vi "Main VI.vi"() -> ()   [LabVIEW 2016]
doc: "Tile child windows in MDI panel"
uses:
  source code/MDI Library/TypeDefs/Set Position.ctl
  Typedef/Queue Operation.ctl
  Typedef/Main VI Data Cluster.ctl
  source code/MDI Library/LV MDI.lvclass
  source code/Document/Document.lvclass
  <vilib>/Utility/error.llb/DialogType.ctl
  source code/MDI Library/Public/Create.vi
  source code/MDI Library/Public/Add.vi
  source code/MDI Library/Public/Remove.vi
  source code/MDI Library/Public/Set Position.vi
  source code/MDI Library/Public/Show.vi
  source code/MDI Library/Public/Hide.vi
  source code/MDI Library/Public/Save.vi
  source code/MDI Library/Public/Recall.vi
  source code/MDI Library/Public/Dock.vi
  source code/MDI Library/Public/Tile.vi
  source code/MDI Library/Public/Cascade.vi
  source code/MDI Library/Public/Destroy.vi
  user32.dll
  System.Windows.Forms
  source code/Document/Child Classes/Py Doc/Py Doc.lvclass
  source code/Document/Child Classes/LV Doc/Child Classes/LV DEV/LV DEV.lvclass
panel:
  in  "Py File Path":path
  in  "XML File Path":path
  in  "Recall":bool
  in  "Save":bool
  in  "Position[]":T1[](array[typedef]) caption="Set Position for selected Documents"
  in  "Remove":bool
  in  "Cascade & Order":cluster{"Order":u16, "Cascade":bool}={"Order"=2, "Cascade"=FALSE} {"Order" items=["List order"=2, "Z order"=4]}
  in  "Tile & Direction":cluster{"Direction":u16, "Tile":bool} {"Direction" items=["Vertical", "Horizontal"]}
  in  "Listbox":i32[](listbox)
  in  "Undock":bool
  in  "Add":bool
  in  "Hide":bool
  in  "Show":bool
  in  "Stop":bool
  in  "LV Dev Path":path
  in  "Container":refnum<k24>(container)
  out "Error Out":errorcluster
  in  "Error In":errorcluster
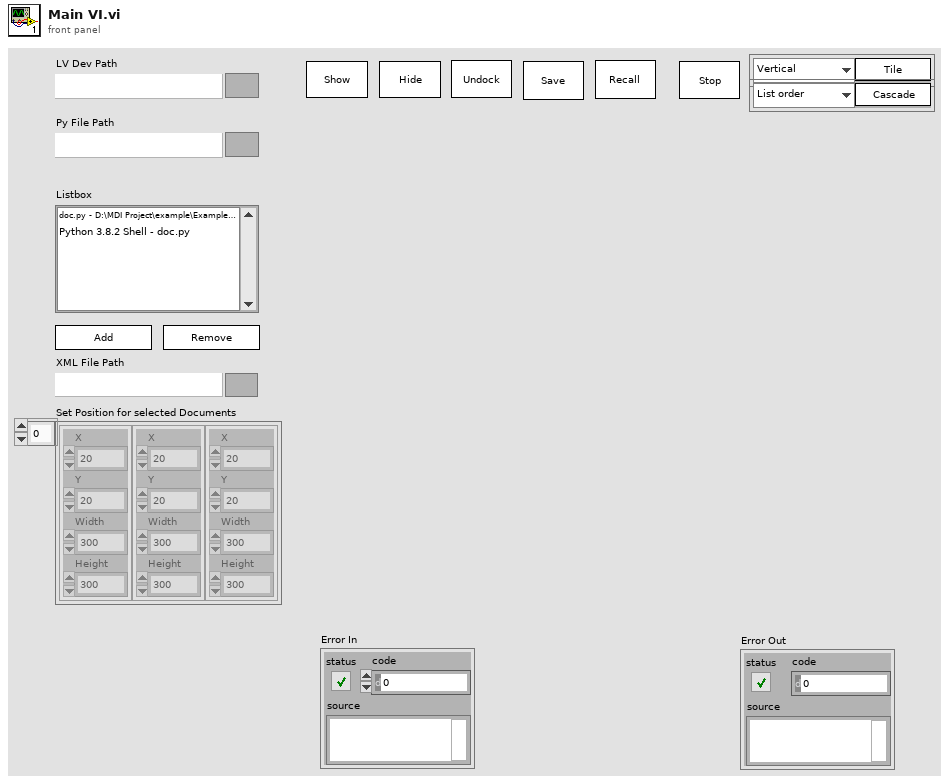
[diagram p1: front panel]
types:
  T1 = typedef "LV MDI.lvclass/Set Position.ctl" = cluster{"X":i32, "Y":i32, "Width":i32, "Height":i32}
  T2 = typedef "Queue Operation.ctl" = enum16{"Create Queue", "Enqueue N Element", "Enstack N Element", "Dequeue 1 Element", "Flush Queue", "Close Queue"}
  T3 = typedef "Main VI Data Cluster.ctl" = cluster{"MDI Object":refnum<class "LV MDI.lvclass">, "Container Refnum":refnum<k24>, "LV Dev  Path":path, "Document Name[]":string[], "LV hwnd":u32, "Dock?":bool, "Position[] ":T1[], "XML File Path ":path, "Document Class":refnum<class "Document.lvclass">, "Py file Path":path, "Document Class[]":refnum<class "Document.lvclass">[]}
  T4 = typedef "DialogType.ctl" = u16
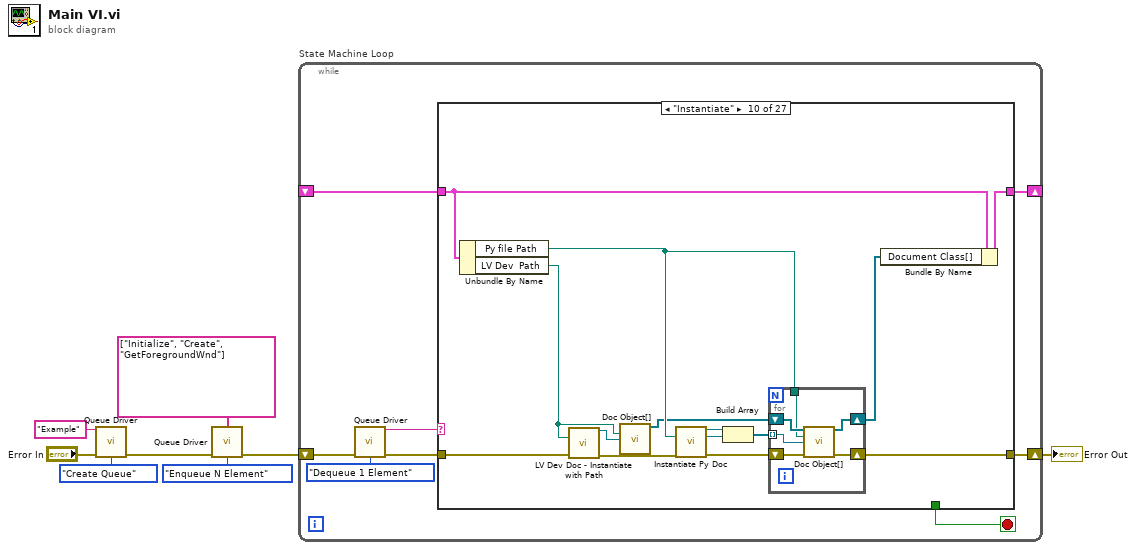
[diagram p0: block diagram]
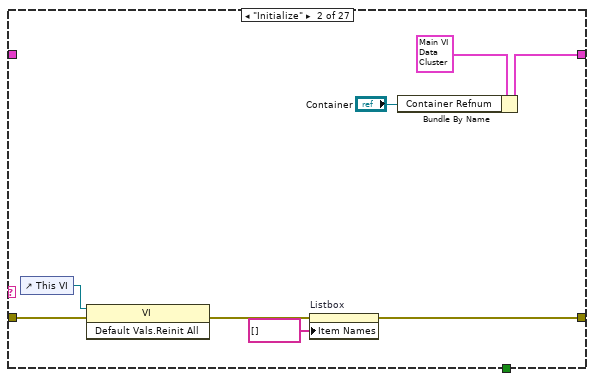
[diagram p3: hidden frame]
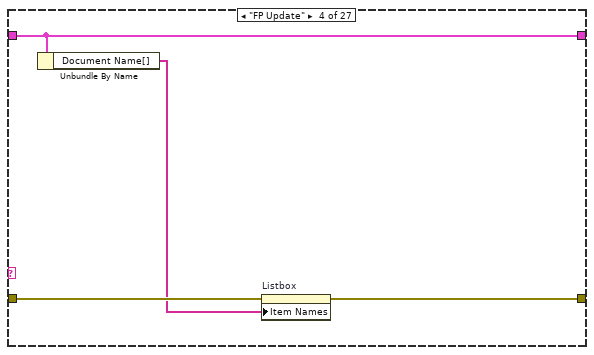
[diagram p5: hidden frame]
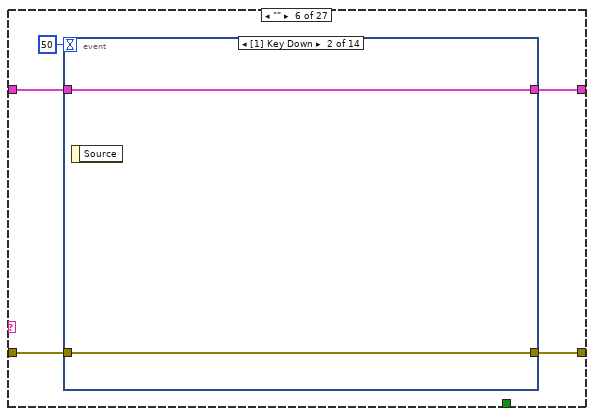
[diagram p7: hidden frame]
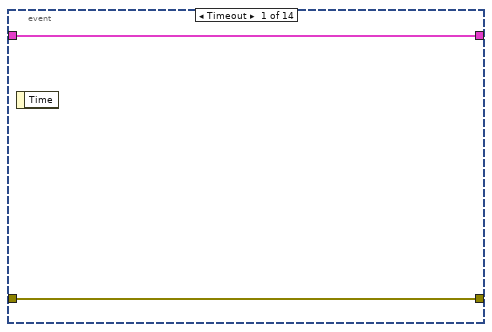
[diagram p8: hidden frame]
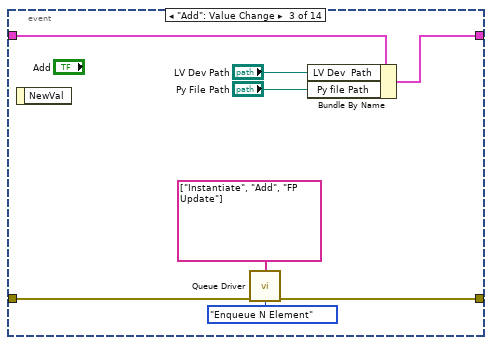
[diagram p9: hidden frame]
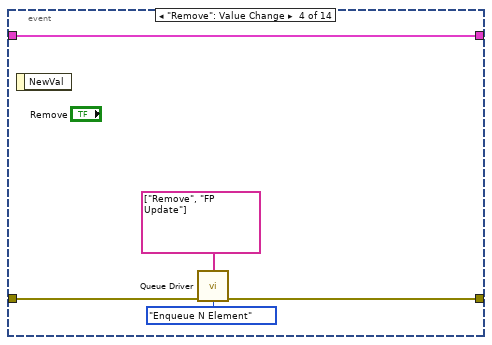
[diagram p10: hidden frame]
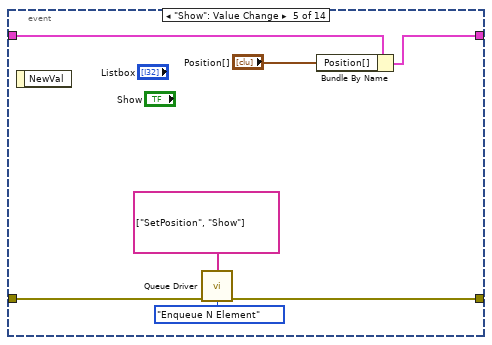
[diagram p11: hidden frame]
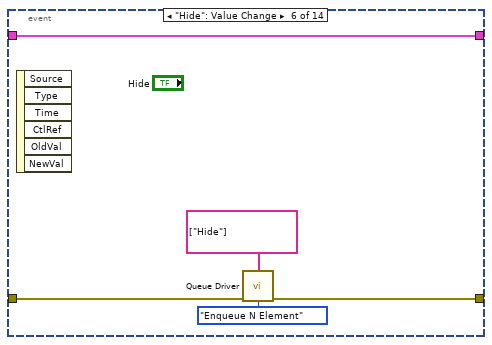
[diagram p12: hidden frame]
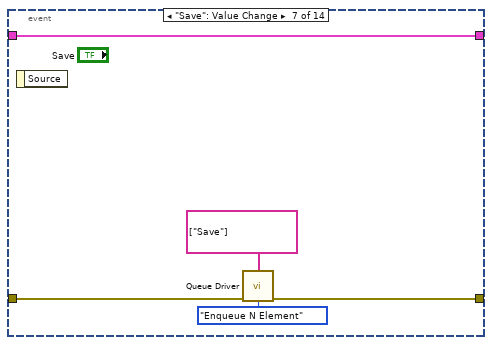
[diagram p13: hidden frame]
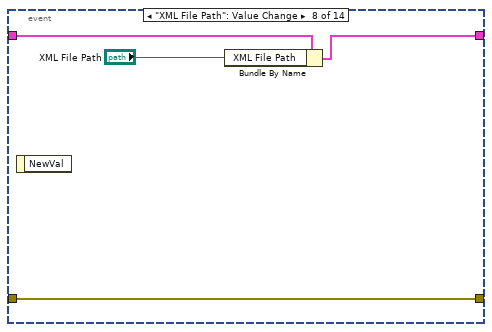
[diagram p14: hidden frame]
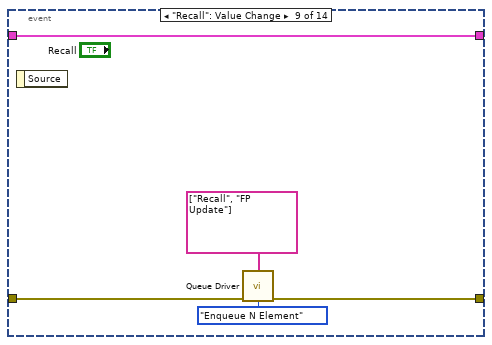
[diagram p15: hidden frame]
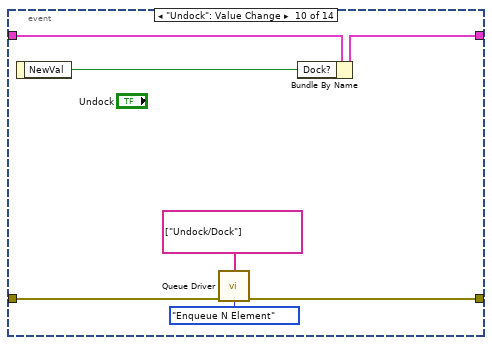
[diagram p16: hidden frame]
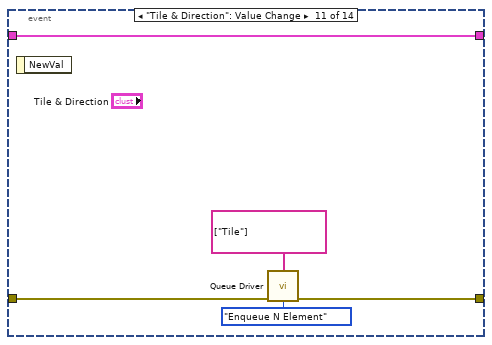
[diagram p17: hidden frame]
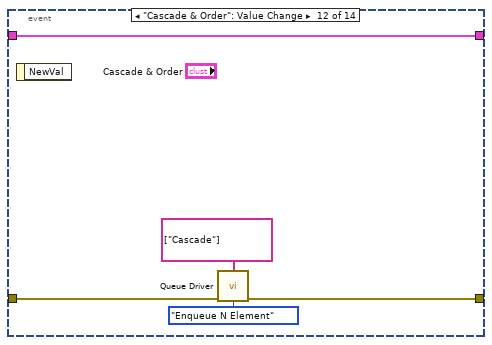
[diagram p18: hidden frame]
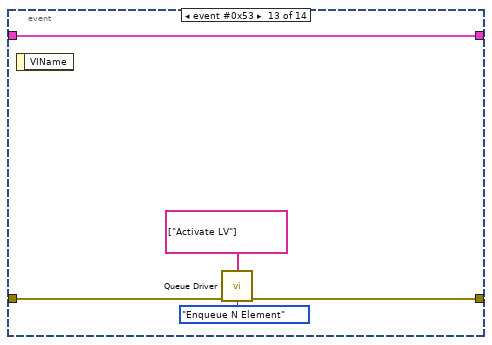
[diagram p19: hidden frame]
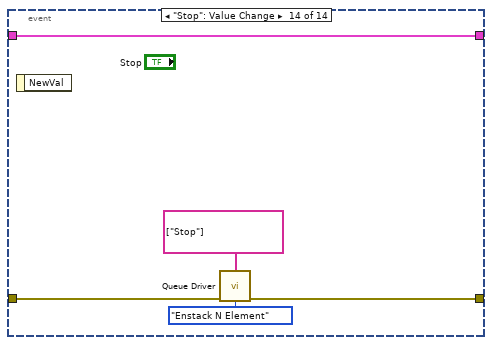
[diagram p20: hidden frame]
diagram:
  n1 = call "Queue Driver.vi"("Queue Name"="Example", "error In"="Error In", "Queue Operation"=Queue_Operation."Create Queue") -> ("error out"=w6:errorcluster)  [unwired: 11 in, 1 out]
  n2 = call "Queue Driver.vi"("States[]"=string[] ["Initialize", "Create", "GetForegroundWnd"], "error In"=w6, "Queue Operation"=Queue_Operation."Enqueue N Element") -> ("error out"=w3:errorcluster)  [unwired: 11 in, 1 out]
  n3 = while "State Machine Loop" {
    shift-right: [w15] -> w7
    shift-left: w3 -> [w16]
    shift-right: [w10] -> _
    shift-left: _ -> [w9]
    stop <- w11 stop-if-true
    n4 = call "Queue Driver.vi"("error In"=w16, "Queue Operation"=Queue_Operation."Dequeue 1 Element") -> ("Dequeued State"=w12:string, "error out"=w14:errorcluster)  [unwired: 12 in]
    n5 = case shown="\"Instantiate\"" w12 {
      selector: w12 -> [_ _ _ _ _ _ _ _ _ _ _ _ _ _ _ _ _ _ _ _ _ _ _ _ w258 _ _]
      tunnel: w14 -> [w18 w26 w28 w32 w34 w39 w111 w118 w123 w128 w149 w167 w172 w186 w190 w202 w209 w221 w223 w231 w239 w241 w245 w251 w259 w272 w284]
      tunnel: [w18 w20 w28 w31 w34 w38 w111 w117 w122 w134 w148 w161 w177 w185 w195 w201 w208 w220 w223 w230 w238 w241 w244 w251 w255 w262 w290] -> w15
      tunnel: [_ _ _ _ _ _ _ _ _ _ _ _ _ _ _ _ _ _ _ _ _ _ _ _ _ _ TRUE] -> w11
      tunnel: [w17 w24 w27 w30 w33 w35 w110 w114 w120 w136 w150 w164 w174 w181 w192 w198 w210 w217 w222 w226 w234 w240 w243 w250 w252 w260 w287] -> w10
      tunnel: w9 -> [w17 _ w27 w30 w33 w36 w110 w115 w121 w137 w151 w165 w175 w182 w193 w199 w211 w218 w222 w227 w235 w240 w243 w250 w252 w260 w288]
      frame "----------------------Initialization---------------------" {
      }
      frame "Initialize" {
        n6 = control-ref of="This VI"() -> (w21:refnum<vi>)
        n7 = invoke class="VI" method="Default Vals.Reinit All"(reference=w21, error in=w26) -> (error out=w22:errorcluster)  [unwired: 1 in, 2 out]
        n8 = property on="Listbox" class="LstBox (strict)"(error in=w22, "Item Names"=string[] []) -> (error out=w20:errorcluster)  [unwired: 1 in, 1 out]
        n9 = Bundle By Name(cluster=T3 {"MDI Object"=refnum, "Container Refnum"=refnum, "LV Dev  Path"=path "", "Document Name[]"=[], "LV hwnd"=0, "Dock?"=FALSE, "Position[] "=[], "XML File Path "=path "", "Document Class"=refnum, "Py file Path"=path "", "Document Class[]"=[]}, "Container Refnum"="Container") -> (w24:T3)
      }
      frame "----------------------Front Panel Update-------------" {
      }
      frame "FP Update" {
        n10 = Unbundle By Name(w30) -> ("Document Name[]"=w29:string[])
        n11 = property on="Listbox" class="LstBox (strict)"(error in=w32, "Item Names"=w29) -> (error out=w31:errorcluster)  [unwired: 1 in, 1 out]
      }
      frame "----------------------Poll-------------------------------" {
      }
      frame "" {
        n12 = event shown="[1] Key Down" {
          selector: _ -> [_ _ _ _ _ _ _ _ _ _ _ _ _ _]
          dyn-events: _ -> [_ _ _ _ _ _ _ _ _ _ _ _ _ _]
          timeout: 50 -> [_ _ _ _ _ _ _ _ _ _ _ _ _ _]
          tunnel: [w41 w43 w47 w54 w62 w66 w72 w77 w80 w88 w92 w97 w102 w107] -> w38
          tunnel: w39 -> [w41 w43 w51 w56 w63 w68 w73 w77 w82 w89 w94 w99 w104 w109]
          tunnel: [w40 w42 w48 w55 w58 w67 w69 w75 w81 w84 w93 w98 w103 w108] -> w35
          tunnel: w36 -> [w40 w42 w49 w55 w59 w67 w69 w76 w81 w85 w93 w98 w103 w108]
          event Timeout {
            n13 = event-data() -> ()  [unwired: 1 in, 1 out]
          }
          event Key Down {
            n14 = event-data() -> ()  [unwired: 1 in, 1 out]
          }
          event "Add": Value Change {
            n15 = event-data() -> ()  [unwired: 1 in, 1 out]
            n16 = call "Queue Driver.vi"("States[]"=string[] ["Instantiate", "Add", "FP Update"], "error In"=w51, "Queue Operation"=Queue_Operation."Enqueue N Element") -> ("error out"=w47:errorcluster)  [unwired: 11 in, 1 out]
            n17 = Bundle By Name(cluster=w49, "LV Dev  Path"="LV Dev Path", "Py file Path"="Py File Path") -> (w48:T3)
          }
          event "Remove": Value Change {
            n18 = event-data() -> ()  [unwired: 1 in, 1 out]
            n19 = call "Queue Driver.vi"("States[]"=string[] ["Remove", "FP Update"], "error In"=w56, "Queue Operation"=Queue_Operation."Enqueue N Element") -> ("error out"=w54:errorcluster)  [unwired: 11 in, 1 out]
          }
          event "Show": Value Change {
            n20 = event-data() -> ()  [unwired: 1 in, 1 out]
            n21 = call "Queue Driver.vi"("States[]"=string[] ["SetPosition", "Show"], "error In"=w63, "Queue Operation"=Queue_Operation."Enqueue N Element") -> ("error out"=w62:errorcluster)  [unwired: 11 in, 1 out]
            n22 = Bundle By Name(cluster=w59, "Position[]"="Position[]") -> (w58:T3)
          }
          event "Hide": Value Change {
            n23 = event-data() -> ()  [unwired: 1 in, 6 out]
            n24 = call "Queue Driver.vi"("States[]"=string[] ["Hide"], "error In"=w68, "Queue Operation"=Queue_Operation."Enqueue N Element") -> ("error out"=w66:errorcluster)  [unwired: 11 in, 1 out]
          }
          event "Save": Value Change {
            n25 = event-data() -> ()  [unwired: 1 in, 1 out]
            n26 = call "Queue Driver.vi"("States[]"=string[] ["Save"], "error In"=w73, "Queue Operation"=Queue_Operation."Enqueue N Element") -> ("error out"=w72:errorcluster)  [unwired: 11 in, 1 out]
          }
          event "XML File Path": Value Change {
            n27 = event-data() -> ()  [unwired: 1 in, 1 out]
            n28 = Bundle By Name(cluster=w76, "XML File Path"="XML File Path") -> (w75:T3)
          }
          event "Recall": Value Change {
            n29 = event-data() -> ()  [unwired: 1 in, 1 out]
            n30 = call "Queue Driver.vi"("States[]"=string[] ["Recall", "FP Update"], "error In"=w82, "Queue Operation"=Queue_Operation."Enqueue N Element") -> ("error out"=w80:errorcluster)  [unwired: 11 in, 1 out]
          }
          event "Undock": Value Change {
            n31 = event-data() -> ("NewVal"=w83:bool)  [unwired: 1 in]
            n32 = call "Queue Driver.vi"("States[]"=string[] ["Undock/Dock"], "error In"=w89, "Queue Operation"=Queue_Operation."Enqueue N Element") -> ("error out"=w88:errorcluster)  [unwired: 11 in, 1 out]
            n33 = Bundle By Name(cluster=w85, "Dock?"=w83) -> (w84:T3)
          }
          event "Tile & Direction": Value Change {
            n34 = event-data() -> ()  [unwired: 1 in, 1 out]
            n35 = call "Queue Driver.vi"("States[]"=string[] ["Tile"], "error In"=w94, "Queue Operation"=Queue_Operation."Enqueue N Element") -> ("error out"=w92:errorcluster)  [unwired: 11 in, 1 out]
          }
          event "Cascade & Order": Value Change {
            n36 = event-data() -> ()  [unwired: 1 in, 1 out]
            n37 = call "Queue Driver.vi"("States[]"=string[] ["Cascade"], "error In"=w99, "Queue Operation"=Queue_Operation."Enqueue N Element") -> ("error out"=w97:errorcluster)  [unwired: 11 in, 1 out]
          }
          event event #0x53 {
            n38 = event-data() -> ()  [unwired: 1 in, 1 out]
            n39 = call "Queue Driver.vi"("States[]"=string[] ["Activate LV"], "error In"=w104, "Queue Operation"=Queue_Operation."Enqueue N Element") -> ("error out"=w102:errorcluster)  [unwired: 11 in, 1 out]
          }
          event "Stop": Value Change {
            n40 = event-data() -> ()  [unwired: 1 in, 1 out]
            n41 = call "Queue Driver.vi"("States[]"=string[] ["Stop"], "error In"=w109, "Queue Operation"=Queue_Operation."Enstack N Element") -> ("error out"=w107:errorcluster)  [unwired: 11 in, 1 out]
          }
        }
      }
      frame "----------------------MDI API-------------------------" {
      }
      frame "Create" {
        n42 = Unbundle By Name(w115) -> ("MDI Object"=w116:refnum<class "LV MDI.lvclass">, "Container Refnum"=w112:refnum<k24>)
        n43 = call-poly "MDI.vi"("LV MDI in"=w116, "Panel Reference"=w112, "error in (no error)"=w118) -> ("LV MDI out"=w113:refnum<class "LV MDI.lvclass">, "error out"=w117:errorcluster)  [unwired: 11 in]
        n44 = Bundle By Name(cluster=w115, "MDI Object"=w113) -> (w114:T3)
      }
      frame "GetForegroundWnd" {
        n45 = dll-call lib="user32.dll" fn="GetForegroundWindow"(error in=w123) -> (error out=w122:errorcluster, "hwnd"=w119:u32)  [unwired: 2 in, 1 out]
        n46 = Bundle By Name(cluster=w121, "LV hwnd"=w119) -> (w120:T3)
      }
      frame "Instantiate" {
        n47 = Unbundle By Name(w137) -> ("Py file Path"=w132:path, "LV Dev  Path"=w124:path)
        n48 = call "LV Dev Doc - Instantiate with Path.vi"("LV Doc Path"=w124, "error in (no error)"=w128) -> ("Document out"=w125:refnum<class "Document.lvclass">, "error out"=w127:errorcluster)  [unwired: 12 in]
        n49 = call "Doc Object[].vi"("Path"=w124, "Document Class"=w125) -> ("Document Class[]"=w126:refnum<class "Document.lvclass">[])  [unwired: 12 in, 1 out]
        n50 = call "Instantiate Py Doc.vi"("Py File Path"=w132, "error in (no error)"=w127) -> ("Editor Document"=w131:refnum<class "Document.lvclass">, "Shell Document"=w130:refnum<class "Document.lvclass">, "error out"=w133:errorcluster)  [unwired: 11 in]
        n51 = Build Array(w131, w130) -> (w129:refnum<class "Document.lvclass">[])
        n52 = for {
          tunnel: w132 -> [w139]
          shift-right: [w143] -> w135
          shift-left: w126 -> [w142]
          shift-right: [w141] -> w134
          shift-left: w133 -> [w140]
          tunnel: w129 -> [w138] mode=indexing
          n53 = call "Doc Object[].vi"("Document Class[]"=w142, "Path"=w139, "Document Class"=w138, "error in (no error)"=w140) -> ("Document Class[]"=w143:refnum<class "Document.lvclass">[], "error out"=w141:errorcluster)  [unwired: 10 in]
        }
        n54 = Bundle By Name(cluster=w137, "Document Class[]"=w135) -> (w136:T3)
      }
      frame "Add" {
        n55 = Unbundle By Name(w151) -> ("MDI Object"=w147:refnum<class "LV MDI.lvclass">, "Document Class[]"=w144:refnum<class "Document.lvclass">[])
        n56 = for {
          tunnel: [w153] -> w145
          shift-right: [w156] -> w148
          shift-left: w149 -> [w157]
          shift-right: [w154] -> w146
          shift-left: w147 -> [w155]
          tunnel: w144 -> [w152] mode=indexing
          n57 = call-poly "MDI.vi"("LV MDI.lvclass"=w155, "Document class"=w152, "error in (no error)"=w157) -> ("LV MDI.lvclass"=w154:refnum<class "LV MDI.lvclass">, "Name[]"=w153:string[], "error out"=w156:errorcluster)  [unwired: 10 in]
        }
        n58 = Bundle By Name(cluster=w151, "MDI Object"=w146, "Document Name[]"=w145) -> (w150:T3)
      }
      frame "Remove" {
        n59 = Unbundle By Name(w165) -> ("MDI Object"=w166:refnum<class "LV MDI.lvclass">)
        n60 = control-ref of="Listbox"() -> (w159:refnum<vi>)
        n61 = call "Selected Doc Name[].vi"("error in (no error)"=w167, "ListBox in"=w159) -> ("error out"=w162:errorcluster, "Array"=w160:string[])  [unwired: 8 in]
        n62 = call-poly "MDI.vi"("LV MDI in"=w166, "Doc Name[]"=w160, "error in (no error)"=w162) -> ("LV MDI out"=w163:refnum<class "LV MDI.lvclass">, "Doc Name out[]"=w158:string[], "error out"=w161:errorcluster)  [unwired: 10 in]
        n63 = Bundle By Name(cluster=w165, "MDI Object"=w163, "Document Name[]"=w158) -> (w164:T3)
      }
      frame "SetPosition" {
        n64 = control-ref of="Listbox"() -> (w169:refnum<vi>)
        n65 = Unbundle By Name(w175) -> ("MDI Object"=w176:refnum<class "LV MDI.lvclass">, "Position[]"=w168:T1[])
        n66 = call "Selected Doc Name[].vi"("error in (no error)"=w172, "ListBox in"=w169) -> ("error out"=w171:errorcluster, "Array"=w170:string[])  [unwired: 8 in]
        n67 = call-poly "MDI.vi"("LV MDI.lvclass"=w176, "Position[]"=w168, "Doc Name[]"=w170, "error in (no error)"=w171) -> ("LV MDI.lvclass"=w173:refnum<class "LV MDI.lvclass">, "error out"=w177:errorcluster)  [unwired: 10 in]
        n68 = Bundle By Name(cluster=w175, "MDI Object"=w173) -> (w174:T3)
      }
      frame "Show" {
        n69 = control-ref of="Listbox"() -> (w178:refnum<vi>)
        n70 = Unbundle By Name(w182) -> ("MDI Object"=w184:refnum<class "LV MDI.lvclass">)
        n71 = call "Selected Doc Name[].vi"("error in (no error)"=w186, "ListBox in"=w178) -> ("error out"=w180:errorcluster, "Array"=w179:string[])  [unwired: 8 in]
        n72 = call-poly "MDI.vi"("LV MDI in"=w184, "Doc Name[]"=w179, "error in (no error)"=w180) -> ("LV MDI out"=w183:refnum<class "LV MDI.lvclass">, "error out"=w185:errorcluster)  [unwired: 11 in]
        n73 = Bundle By Name(cluster=w182, "MDI Object"=w183) -> (w181:T3)
      }
      frame "Hide" {
        n74 = control-ref of="Listbox"() -> (w187:refnum<vi>)
        n75 = Unbundle By Name(w193) -> ("MDI Object"=w194:refnum<class "LV MDI.lvclass">)
        n76 = call "Selected Doc Name[].vi"("error in (no error)"=w190, "ListBox in"=w187) -> ("error out"=w189:errorcluster, "Array"=w188:string[])  [unwired: 8 in]
        n77 = call-poly "MDI.vi"("LV MDI in"=w194, "Doc Name[]"=w188, "error in (no error)"=w189) -> ("LV MDI out"=w191:refnum<class "LV MDI.lvclass">, "error out"=w195:errorcluster)  [unwired: 11 in]
        n78 = Bundle By Name(cluster=w193, "MDI Object"=w191) -> (w192:T3)
      }
      frame "Save" {
        n79 = Unbundle By Name(w199) -> ("MDI Object"=w200:refnum<class "LV MDI.lvclass">, "XML File Path"=w196:path)
        n80 = call-poly "MDI.vi"("LV MDI in"=w200, "XML File Path"=w196, "error in (no error)"=w202) -> ("LV MDI out"=w197:refnum<class "LV MDI.lvclass">, "error out"=w201:errorcluster)  [unwired: 11 in]
        n81 = Bundle By Name(cluster=w199, "MDI Object"=w197) -> (w198:T3)
      }
      frame "Recall" {
        n82 = Unbundle By Name(w211) -> ("MDI Object"=w206:refnum<class "LV MDI.lvclass">, "XML File Path"=w205:path, "Container Refnum"=w204:refnum<k24>)
        n83 = call-poly "MDI.vi"("LV MDI in"=w206, "XML File Path"=w205, "Container Refnum"=w204, "error in (no error)"=w209) -> ("LV MDI out"=w207:refnum<class "LV MDI.lvclass">, "Name[]"=w203:string[], "error out"=w208:errorcluster)  [unwired: 9 in]
        n84 = Bundle By Name(cluster=w211, "MDI Object"=w207, "Document Name[]"=w203) -> (w210:T3)
      }
      frame "Undock/Dock" {
        n85 = control-ref of="Listbox"() -> (w212:refnum<vi>)
        n86 = Unbundle By Name(w218) -> ("MDI Object"=w219:refnum<class "LV MDI.lvclass">, "Dock?"=w215:bool)
        n87 = call "Selected Doc Name[].vi"("error in (no error)"=w221, "ListBox in"=w212) -> ("error out"=w214:errorcluster, "Array"=w213:string[])  [unwired: 8 in]
        n88 = call-poly "MDI.vi"("LV MDI.lvclass"=w219, "Undock?"=w215, "Doc Name[]"=w213, "error in (no error)"=w214) -> ("LV MDI.lvclass"=w216:refnum<class "LV MDI.lvclass">, "error out"=w220:errorcluster)  [unwired: 10 in]
        n89 = Bundle By Name(cluster=w218, "MDI Object"=w216) -> (w217:T3)
      }
      frame "---------------------Styles----------------------------" {
      }
      frame "Tile" {
        n90 = property on="Direction" class="Ring (strict)"(error in=w231) -> (error out=w229:errorcluster, "Value"=w228:u16)  [unwired: 1 in, 1 out]
        n91 = Unbundle By Name(w227) -> ("MDI Object"=w225:refnum<class "LV MDI.lvclass">)
        n92 = call-poly "MDI.vi"("LV MDI.lvclass"=w225, "Tile Direction"=w228, "error in (no error)"=w229) -> ("LV MDI.lvclass"=w224:refnum<class "LV MDI.lvclass">, "error out"=w230:errorcluster)  [unwired: 11 in]
        n93 = Bundle By Name(cluster=w227, "MDI Object"=w224) -> (w226:T3)
      }
      frame "Cascade" {
        n94 = Unbundle By Name(w235) -> ("MDI Object"=w233:refnum<class "LV MDI.lvclass">)
        n95 = property on="Order" class="Ring (strict)"(error in=w239) -> (error out=w237:errorcluster, "Value"=w236:u16)  [unwired: 1 in, 1 out]
        n96 = call-poly "MDI.vi"("LV MDI in"=w233, "Order"=w236, "error in (no error)"=w237) -> ("LV MDI out"=w232:refnum<class "LV MDI.lvclass">, "error out"=w238:errorcluster)  [unwired: 11 in]
        n97 = Bundle By Name(cluster=w235, "MDI Object"=w232) -> (w234:T3)
      }
      frame "---------------------Click-Through--------------------" {
      }
      frame "Activate LV" {
        n98 = Unbundle By Name(w243) -> ("LV hwnd"=w242:u32)
        n99 = disable-structure shown="Disabled" {
          disable-tunnel: w245 -> [w248 w249]
          disable-tunnel: [w247 w249] -> w244
          disable-tunnel: w242 -> [w246 _]
          frame Disabled {
            n100 = call "Drop Through Click.vi"("error in (no error)"=w248, "hwnd"=w246) -> ("error out"=w247:errorcluster)  [unwired: 9 in]
          }
          frame Enabled {
          }
        }
      }
      frame "---------------------Miscellaneous---------------------" {
      }
      frame Default {
        n101 = Concatenate Strings(w258, " State is not found" ("string")) -> (w256:string)
        n102 = One Button Dialog(message=w256) -> ()  [unwired: 1 in, 1 out]
        n103 = call "Queue Driver.vi"("States[]"=string[] ["Stop"], "error In"=w259, "Queue Operation"=Queue_Operation."Enstack N Element") -> ("error out"=w255:errorcluster)  [unwired: 11 in, 1 out]
      }
      frame "Error Handler" {
        w270 = T4 0 items=["no dialog", "OK message", "continue or stop message", "OK message + warnings", "continue/stop + warnings"] ("type of dialog (OK msg:1)")
        n104 = call <vilib>:"Simple Error Handler.vi"("type of dialog (OK msg:1)"=w270, "error in (no error)"=w272) -> ("source out"=w267:string, "error out"=w271:errorcluster)  [unwired: 3 in, 3 out]
        n105 = call <vilib>:"Clear Errors.vi"("error in (no error)"=w271) -> ("error out"=w269:errorcluster)  [unwired: 5 in, 1 out]
        n106 = Format Into String(error in=w269, w267, "\r\n", "Do you wish to continue?" ("input 3")) -> (resulting string=w264:string, error out=w268:errorcluster)  [unwired: 2 in]
        n107 = Two Button Dialog(message=w264, 1:"Abort" ("F button name (\"Cancel\")")) -> (T button?=w261:bool)  [unwired: 1 in]
        n108 = case shown="False" w261 {
          tunnel: w268 -> [w276 w282]
          tunnel: [w275 w279] -> w262
          frame False {
            n109 = call "Queue Driver.vi"("States[]"=string[] ["Stop"], "error In"=w276, "Queue Operation"=Queue_Operation."Enstack N Element") -> ("error out"=w275:errorcluster)  [unwired: 11 in, 1 out]
          }
          frame True {
            n110 = call "Queue Driver.vi"("error In"=w282, "Queue Operation"=Queue_Operation."Flush Queue") -> ("error out"=w281:errorcluster)  [unwired: 12 in, 1 out]
            n111 = call "Queue Driver.vi"("States[]"=string[] ["Initialize"], "error In"=w281, "Queue Operation"=Queue_Operation."Enqueue N Element") -> ("error out"=w279:errorcluster)  [unwired: 11 in, 1 out]
          }
        }
      }
      frame "Stop" {
        n112 = Unbundle By Name(w288) -> ("MDI Object"=w286:refnum<class "LV MDI.lvclass">)
        n113 = call-poly "MDI.vi"("LV MDI in"=w286, "error in (no error)"=w284) -> ("LV MDI out"=w285:refnum<class "LV MDI.lvclass">, "error out"=w283:errorcluster)  [unwired: 12 in]
        n114 = Bundle By Name(cluster=w288, "MDI Object"=w285) -> (w287:T3)
        n115 = call "Queue Driver.vi"("error In"=w283, "Queue Operation"=Queue_Operation."Flush Queue") -> ("error out"=w292:errorcluster)  [unwired: 12 in, 1 out]
        n116 = call "Queue Driver.vi"("error In"=w292, "Queue Operation"=Queue_Operation."Close Queue") -> ("error out"=w290:errorcluster)  [unwired: 12 in, 1 out]
      }
    }
  }
  "Error Out" <- w7
